vi "XMLUpdateHeaders.vi"(10 "#Columns":i32, 11 "TableHeaderIn":string) -> (3 "TableHeaderOut":string)   [LabVIEW 2014]
uses:
  <vilib>/regexp/Match Regular Expression.xnode
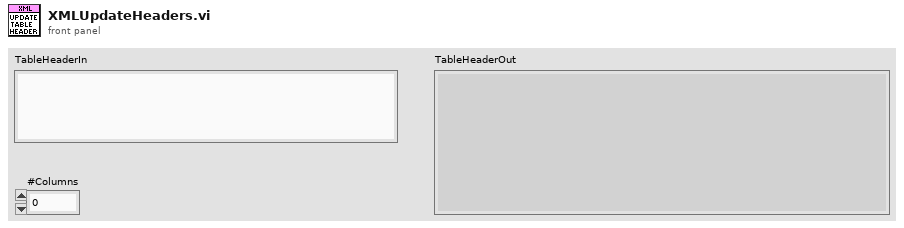
[diagram p1: front panel]
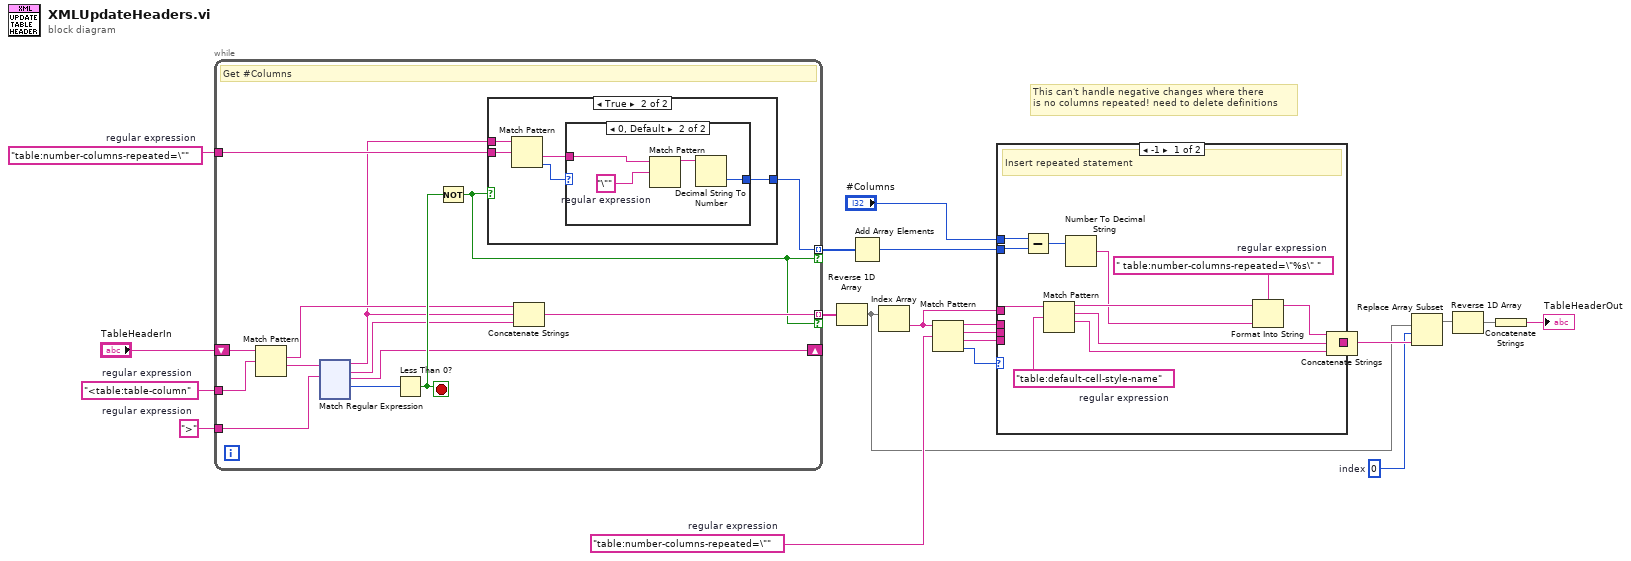
[diagram p0: block diagram]
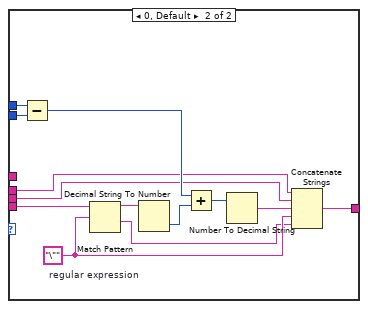
[diagram p2: hidden frame]
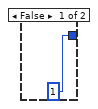
[diagram p3: hidden frame]
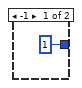
[diagram p4: hidden frame]
diagram:
  w3 = 0  # index
  w14 = "table:number-columns-repeated=\""  # regular expression
  w17 = "table:number-columns-repeated=\""  # regular expression
  w20 = ">"  # regular expression
  w19 = "<table:table-column"  # regular expression
  # "This can't handle negative changes where there\nis no columns repeated! need to delete definitions"
  n1 = while {
    shift-right: [w29] -> _
    shift-left: "TableHeaderIn" -> [w34]
    tunnel: w19 -> [w33]
    tunnel: w20 -> [w30]
    tunnel: [w26] -> w16 mode=indexing if=w21
    tunnel: w17 -> [w27]
    tunnel: [w22] -> w15 mode=indexing if=w21
    stop <- w32 stop-if-true
    # "Get #Columns"
    n2 = Match Pattern(string=w34, regular expression=w33) -> (match substring=w25:string, after substring=w31:string)  [unwired: 1 in, 2 out]
    n3 = xnode "Match Regular Expression"("input string"=w31, "regular expression"=w30) -> ("before match"=w24:string, "whole match"=w23:string, "after match"=w29:string, "offset past match"=w28:i32)  [unwired: 4 in, 1 out]
    n4 = Less Than 0?(x=w28) -> (x < 0?=w32:bool)
    n5 = Not(x=w32) -> (.not. x?=w21:bool)
    n6 = case shown="True" w21 {
      tunnel: w24 -> [_ w40]
      tunnel: w27 -> [_ w39]
      tunnel: [1 w37] -> w26
      frame False {
      }
      frame True {
        n7 = Match Pattern(string=w40, regular expression=w39) -> (after substring=w38:string, offset past match=w36:i32)  [unwired: 1 in, 2 out]
        n8 = case shown="0, Default" w36 {
          tunnel: w38 -> [_ w45]
          tunnel: [1 w42] -> w37
          frame -1 {
          }
          frame 0, Default {
            w44 = "\""  # regular expression
            n9 = Match Pattern(string=w45, regular expression=w44) -> (before substring=w43:string)  [unwired: 1 in, 3 out]
            n10 = Decimal String To Number(string=w43) -> (number=w42:i32)  [unwired: 2 in, 1 out]
          }
        }
      }
    }
    n11 = Concatenate Strings(w25, w24, w23) -> (w22:string)
  }
  n12 = Reverse 1D Array(array=w15) -> (reversed array=w8:string[])
  n13 = Add Array Elements(numeric array=w16) -> (sum=w11:i32)
  n14 = Index Array(array=w8) -> (element=w12:string)  [unwired: 1 in]
  n15 = Match Pattern(string=w12, regular expression=w14) -> (before substring=w5:string, match substring=w4:string, after substring=w13:string, offset past match=w7:i32)  [unwired: 1 in]
  n16 = case shown="-1" w7 {
    tunnel: w13 -> [_ w184]
    tunnel: w12 -> [w170 _]
    tunnel: w11 -> [w166 w181]
    tunnel: "#Columns" -> [w168 w182]
    tunnel: [w160 w175] -> w9
    tunnel: w5 -> [_ w174]
    tunnel: w4 -> [_ w173]
    frame -1 {
      w169 = " table:number-columns-repeated=\"%s\" "  # regular expression
      w171 = "table:default-cell-style-name"  # regular expression
      # "Insert repeated statement"
      n17 = Subtract(x=w168, y=w166) -> (x-y=w165:i32)
      n18 = Match Pattern(string=w170, regular expression=w171) -> (before substring=w167:string, match substring=w162:string, after substring=w161:string)  [unwired: 1 in, 1 out]
      n19 = Number To Decimal String(number=w165) -> (decimal integer string=w164:string)  [unwired: 1 in]
      n20 = Format Into String(format string=w169, initial string=w167, w164) -> (resulting string=w163:string)  [unwired: 1 in, 1 out]
      n21 = Concatenate Strings(w163, w162, w161) -> (w160:string)
    }
    frame 0, Default {
      w176 = "\""  # regular expression
      n22 = Subtract(x=w182, y=w181) -> (x-y=w179:i32)
      n23 = Match Pattern(string=w184, regular expression=w176) -> (before substring=w183:string, after substring=w172:string)  [unwired: 1 in, 2 out]
      n24 = Decimal String To Number(string=w183) -> (number=w180:i32)  [unwired: 2 in, 1 out]
      n25 = Add(x=w179, y=w180) -> (x+y=w178:i32)
      n26 = Number To Decimal String(number=w178) -> (decimal integer string=w177:string)  [unwired: 1 in]
      n27 = Concatenate Strings(w174, w173, w177, w176, w172) -> (w175:string)
    }
  }
  n28 = Replace Array Subset(array=w8, new element=w9, index=w3) -> (w6:string[])
  n29 = Reverse 1D Array(array=w6) -> (reversed array=w2:string[])
  n30 = Concatenate Strings(w2) -> (→"TableHeaderOut":string)
